vi "test.vi"() -> ()   [LabVIEW 2015]
panel:
  out "Waveform Chart":dbl(graph)
  in  "noSteps":i32
  in  "Stop acquisition":bool
  in  "Begin acquisition":bool
  in  "end all comms and exit":bool
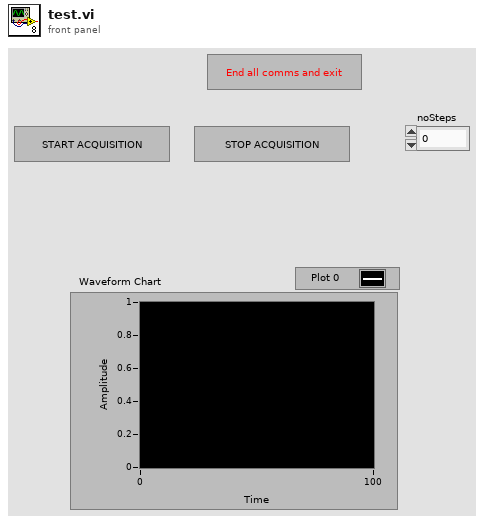
[diagram p1: front panel]
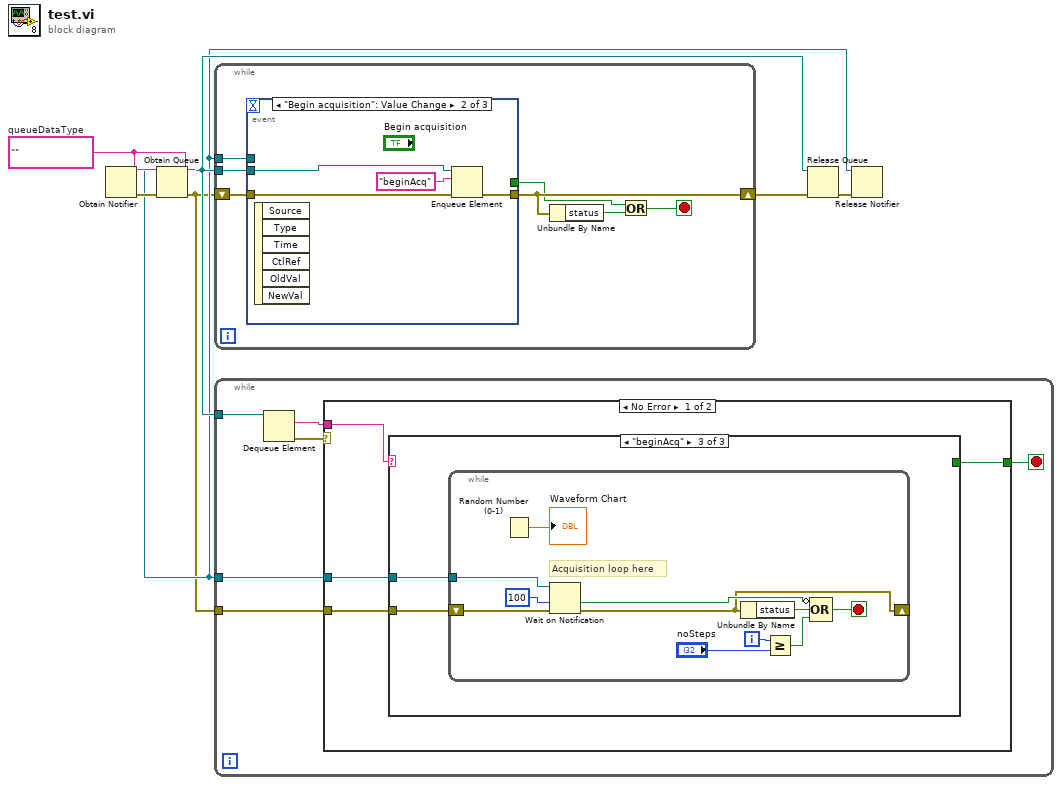
[diagram p0: block diagram]
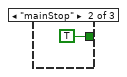
[diagram p3: hidden frame]
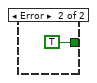
[diagram p4: hidden frame]
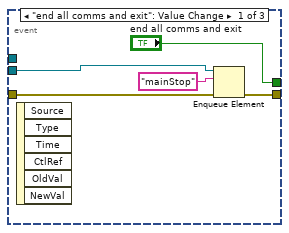
[diagram p5: hidden frame]
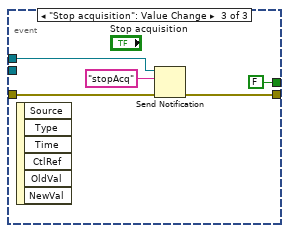
[diagram p6: hidden frame]
diagram:
  w6 = ""  # queueDataType
  n1 = Obtain Notifier(notification data type=w6) -> (notifier out=w2:refnum<notifier>, error out=w7:errorcluster)  [unwired: 3 in, 1 out]
  n2 = Obtain Queue(element data type=w6, error in (no error)=w7) -> (queue out=w3:refnum<queue>, error out=w1:errorcluster)  [unwired: 3 in, 1 out]
  n3 = while {
    shift-right: [w13] -> w5
    shift-left: w1 -> [w14]
    tunnel: w3 -> [w9]
    tunnel: w2 -> [w8]
    stop <- w10 stop-if-true
    n4 = event shown="[1] \"Begin acquisition\": Value Change" {
      selector: _ -> [_ _ _]
      dyn-events: _ -> [_ _ _]
      timeout: _ -> [_ _ _]
      tunnel: ["end all comms and exit" _ FALSE ("end all comms and exit")] -> w11
      tunnel: w14 -> [w18 w21 w26]
      tunnel: [w17 w20 w25] -> w13
      tunnel: w9 -> [w15 w22 _]
      tunnel: w8 -> [_ _ w27]
      event "end all comms and exit": Value Change {
        n5 = event-data() -> ()  [unwired: 1 in, 6 out]
        n6 = Enqueue Element(queue=w15, element="mainStop", error in (no error)=w18) -> (error out=w17:errorcluster)  [unwired: 1 in, 2 out]
      }
      event "Begin acquisition": Value Change {
        n7 = event-data() -> ()  [unwired: 1 in, 6 out]
        n8 = Enqueue Element(queue=w22, element="beginAcq", error in (no error)=w21) -> (error out=w20:errorcluster)  [unwired: 1 in, 2 out]
      }
      event "Stop acquisition": Value Change {
        n9 = event-data() -> ()  [unwired: 1 in, 6 out]
        n10 = Send Notification(notification="stopAcq" ("element"), notifier=w27, error in (no error)=w26) -> (error out=w25:errorcluster)  [unwired: 1 out]
      }
    }
    n11 = Unbundle By Name(w13) -> ("status"=w12:bool)
    n12 = Or(x=w11, y=w12) -> (x .or. y?=w10:bool)
  }
  n13 = while {
    tunnel: w3 -> [w31]
    tunnel: w2 -> [w30]
    tunnel: w1 -> [w29]
    stop <- w32 stop-if-true
    n14 = Dequeue Element(queue=w31) -> (element=w33:string, error out=w34:errorcluster)  [unwired: 2 in, 2 out]
    n15 = case shown="No Error" w34 {
      tunnel: w33 -> [w38 _]
      tunnel: [w37 TRUE] -> w32
      tunnel: w30 -> [w36 _]
      tunnel: w29 -> [w35 _]
      frame No Error {
        n16 = case shown="\"beginAcq\"" w38 {
          tunnel: [_ TRUE _] -> w37
          tunnel: w36 -> [_ _ w41]
          tunnel: w35 -> [_ _ w40]
          frame "False", Default {
          }
          frame "mainStop" {
          }
          frame "beginAcq" {
            n17 = while {
              tunnel: w41 -> [w52]
              shift-right: [w42] -> _
              shift-left: w40 -> [w51]
              i -> [w46]
              stop <- w50 stop-if-true
              # "Acquisition loop here"
              n18 = Random Number (0-1)() -> (number: 0 to 1=→"Waveform Chart":dbl)
              n19 = Wait on Notification(notifier=w52, timeout in ms (-1)=100, error in (no error)=w51) -> (timed out?=w48:bool, error out=w42:errorcluster)  [unwired: 1 in, 2 out]
              n20 = Unbundle By Name(w42) -> ("status"=w49:bool)
              n21 = Greater Or Equal?(x=w46, y="noSteps") -> (x >= y?=w44:bool)
              n22 = Compound Arithmetic op=OR(invert w48, w49, w44) -> (w50:bool)
            }
          }
        }
      }
      frame Error {
      }
    }
  }
  n23 = Release Queue(queue=w3, error in (no error)=w5) -> (error out=w4:errorcluster)  [unwired: 1 in, 2 out]
  n24 = Release Notifier(notifier=w2, error in (no error)=w4) -> ()  [unwired: 1 in, 3 out]
